vi "Host - DO Update.vi"(6 "Operation":enum16{"Init", "Get", "Set"}(ring)=enum."Get", 10 "DO Input":cluster{"Names":string[], "Data":bool[]}[](array[cluster])) -> (2 "DO Out":cluster{"Names":string[], "Data":bool[]}[](array[cluster]))   [LabVIEW 2021]
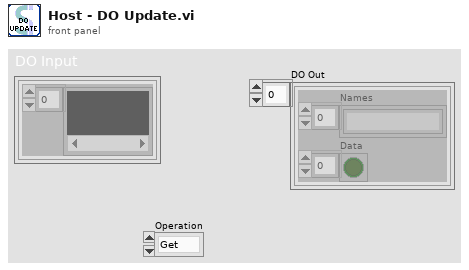
[diagram p1: front panel]
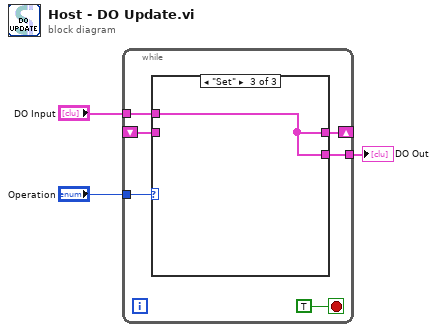
[diagram p0: block diagram]
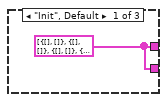
[diagram p2: hidden frame]
diagram:
  n1 = while {
    tunnel: "Operation" -> [w8]
    shift-right: [w7] -> _
    shift-left: _ -> [w6]
    tunnel: [w5] -> w1
    tunnel: "DO Input" -> [w4]
    stop <- TRUE stop-if-true
    n2 = case shown="\"Set\"" w8 {
      tunnel: [w10 w11 w12] -> w7
      tunnel: w6 -> [_ w11 _]
      tunnel: [w10 w11 w12] -> w5
      tunnel: w4 -> [_ _ w12]
      frame "Init", Default {
        w10 = cluster{"Names":string[], "Data":bool[]}[] [{"Names"=[], "Data"=[]}, {"Names"=[], "Data"=[]}, {"Names"=[], "Data"=[]}, {"Names"=[], "Data"=[FALSE, FALSE, FALSE, FALSE, FALSE, FALSE, FALSE, FALSE, FALSE, FALSE, FALSE, FALSE, FALSE, FALSE, FALSE, TRUE]}] ("DO Input")
      }
      frame "Get" {
      }
      frame "Set" {
      }
    }
  }
  "DO Out" <- w1
